vi "Core.vi"() -> ()   [LabVIEW 2020]
uses:
  Standard/Standard.lvclass
  E:/LabVIEW/Actor Learn/LabVIEW Actor Framework/2.Deriving the Actor Core in Actor Framework/Counter/Counter.lvclass
  Complex/Complex.lvclass
  Counter/Counter.lvclass
panel:
  in  "Complex?":bool
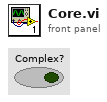
[diagram p1: front panel]
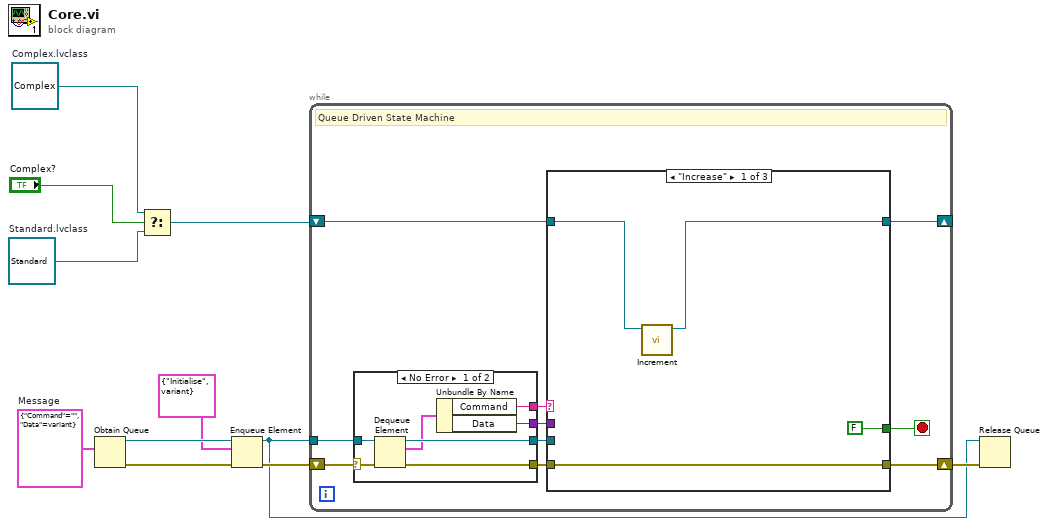
[diagram p0: block diagram]
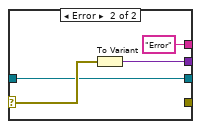
[diagram p2: hidden frame]
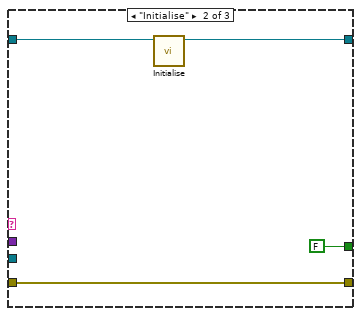
[diagram p3: hidden frame]
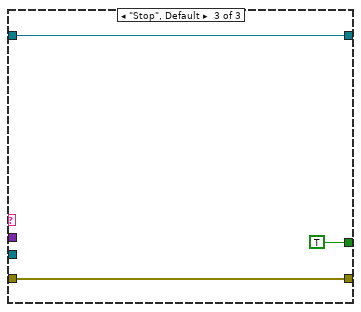
[diagram p4: hidden frame]
diagram:
  w4 = refnum<class "Complex.lvclass"> refnum  # Complex.lvclass
  w3 = refnum<class "Standard.lvclass"> refnum  # Standard.lvclass
  w10 = cluster{"Command":string, "Data":variant} {"Command"="", "Data"=variant}  # Message
  n1 = Obtain Queue(element data type=w10) -> (queue out=w9:refnum<queue>, error out=w8:errorcluster)  [unwired: 4 in, 1 out]
  n2 = Select(t=w4, s="Complex?", f=w3) -> (s? t:f=w2:refnum<class "Counter.lvclass">)
  n3 = Enqueue Element(queue=w9, element=cluster{"Command":string, "Data":variant} {"Command"="Initialise", "Data"=variant}, error in (no error)=w8) -> (queue out=w5:refnum<queue>, error out=w7:errorcluster)  [unwired: 1 in, 1 out]
  n4 = while {
    tunnel: w5 -> [w21]
    shift-right: [w17] -> w11
    shift-left: w7 -> [w20]
    shift-right: [w12] -> _
    shift-left: w2 -> [w13]
    stop <- w14 stop-if-true
    # "Queue Driven State Machine"
    n5 = case shown="No Error" w20 {
      selector: w20 -> [w27 w32]
      tunnel: w21 -> [w28 w29]
      tunnel: [w26 w29] -> w19
      tunnel: [w25 _] -> w18
      tunnel: [w23 "Error" ("Command")] -> w16
      tunnel: [w22 w31] -> w15
      frame No Error {
        n6 = Dequeue Element(queue=w28, error in (no error)=w27) -> (queue out=w26:refnum<queue>, element=w24:cluster{"Command":string, "Data":variant}, error out=w25:errorcluster)  [unwired: 1 in, 1 out]
        n7 = Unbundle By Name(w24) -> ("Command"=w23:string, "Data"=w22:variant)
      }
      frame Error {
        n8 = To Variant(anything=w32) -> (Variant=w31:variant)
      }
    }
    n9 = case shown="\"Increase\"" w16 {
      tunnel: w19 -> [_ _ _]
      tunnel: w18 -> [w36 w40 w43]
      tunnel: [w36 w40 w43] -> w17
      tunnel: w15 -> [_ _ _]
      tunnel: [FALSE FALSE TRUE] -> w14
      tunnel: w13 -> [w34 w38 w41]
      tunnel: [w33 w37 w41] -> w12
      frame "Increase" {
        n10 = call-dynamic "Increment.vi"("Counter in"=w34) -> ("Counter out"=w33:refnum<class "Counter.lvclass">)  [unwired: 9 in, 1 out]
      }
      frame "Initialise" {
        n11 = call-dynamic "Initialise.vi"("Counter in"=w38) -> ("Counter out"=w37:refnum<class "Counter.lvclass">)  [unwired: 9 in, 1 out]
      }
      frame "Stop", Default {
      }
    }
  }
  n12 = Release Queue(queue=w5, error in (no error)=w11) -> ()  [unwired: 1 in, 3 out]
